vi "PhysMon-Send Notifier.vi"(0 "Path":path, 11 "error in (no error)":errorcluster) -> (15 "error out":errorcluster)   [LabVIEW 2020]
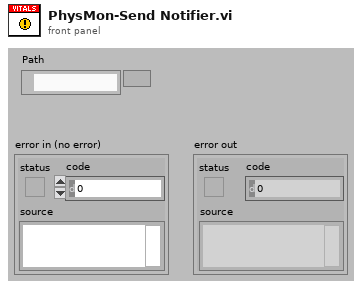
[diagram p1: front panel]
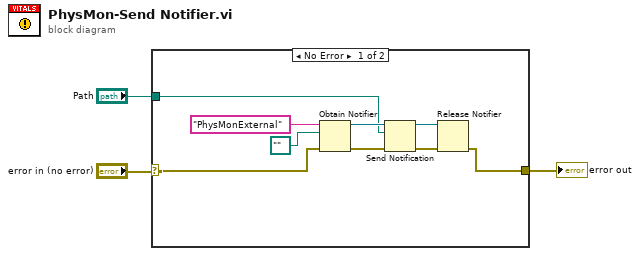
[diagram p0: block diagram]
diagram:
  n1 = case shown="No Error" "error in (no error)" {
    selector: "error in (no error)" -> [w10 w13]
    tunnel: [w4 w13] -> w2
    tunnel: "Path" -> [w7 _]
    frame No Error {
      n2 = Obtain Notifier(name (unnamed)="PhysMonExternal", notification data type=path "" ("File"), error in (no error)=w10) -> (notifier out=w8:refnum<notifier>, error out=w9:errorcluster)  [unwired: 1 in, 1 out]
      n3 = Send Notification(notification=w7, notifier=w8, error in (no error)=w9) -> (notifier out=w5:refnum<notifier>, error out=w6:errorcluster)
      n4 = Release Notifier(notifier=w5, error in (no error)=w6) -> (error out=w4:errorcluster)  [unwired: 1 in, 2 out]
    }
    frame Error {
    }
  }
  "error out" <- w2
